vi "9- Greater than 10 on array of LEDs.vi"() -> ()   [LabVIEW 2019]
panel:
  out "> 10?":bool[](array[boolean])
  out "Array":dbl[](array[numeric])
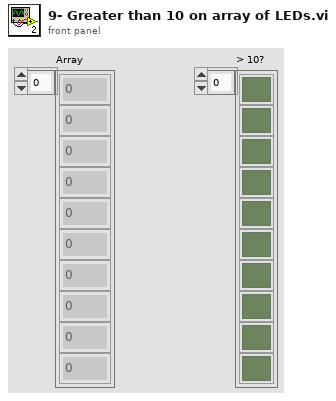
[diagram p1: front panel]
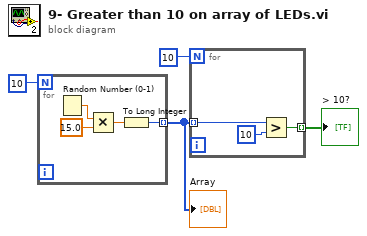
[diagram p0: block diagram]
diagram:
  n1 = for {
    N: 10 -> [_]
    tunnel: [w5] -> w2 mode=indexing
    n2 = Random Number (0-1)() -> (number: 0 to 1=w8:dbl)
    n3 = Multiply(x=w8, y=15.0 ("x*y")) -> (x*y=w6:dbl)
    n4 = To Long Integer(number=w6) -> (32bit integer=w5:i32)
  }
  "Array" <- w2
  n5 = for {
    N: 10 -> [_]
    tunnel: w2 -> [w11] mode=indexing
    tunnel: [w9] -> w1 mode=indexing
    n6 = Greater?(x=w11, y=10) -> (0:w9:bool)
  }
  "> 10?" <- w1
